vi "Map Balloon String.vi"(1 "One more?":bool, 2 "Latitude":dbl format="%#.6g", 3 "character":string, 4 "color":string(combo), 5 "size":string(combo), 6 "Longitude":dbl format="%#.6g") -> (0 "Balloon":string)   [LabVIEW 2011]
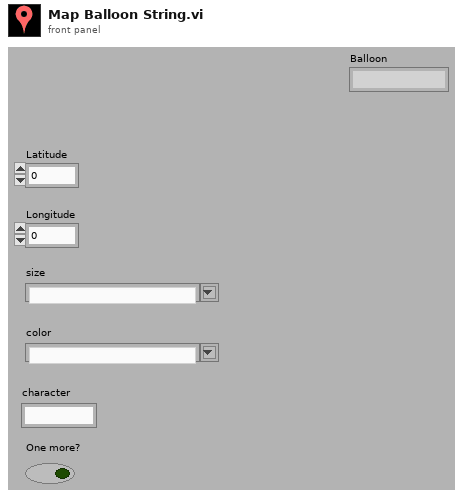
[diagram p1: front panel]
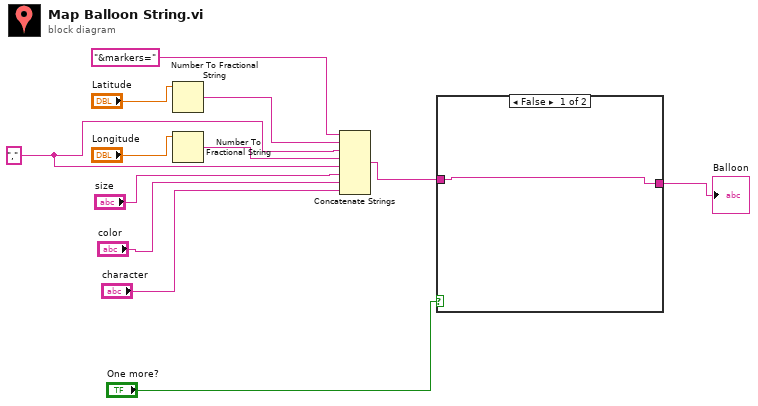
[diagram p0: block diagram]
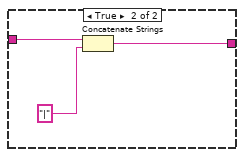
[diagram p2: hidden frame]
diagram:
  w7 = ","
  n1 = Number To Fractional String(number="Latitude") -> (F-format string=w9:string)  [unwired: 3 in]
  n2 = Number To Fractional String(number="Longitude") -> (F-format string=w8:string)  [unwired: 3 in]
  n3 = Concatenate Strings("&markers=", w9, w7, w8, w7, "size", "color", "character") -> (w2:string)
  n4 = case shown="False" "One more?" {
    tunnel: w2 -> [w13 w16]
    tunnel: [w13 w14] -> w1
    frame False {
    }
    frame True {
      n5 = Concatenate Strings(w16, "|") -> (w14:string)
    }
  }
  "Balloon" <- w1
